vi "__FilterSet_CtrlEnable.vi"(4 "EIDRef 2":refnum<vi>[](array[refnum]), 6 "IDRef 2":refnum<vi>[](array[refnum]), 8 "error in (no error)":errorcluster, 9 "EIDRef":refnum<vi>[](array[refnum]), 10 "IDRef":refnum<vi>[](array[refnum]), 11 "CtrlRef":T1) -> (0 "error out":errorcluster)   [LabVIEW 2011]
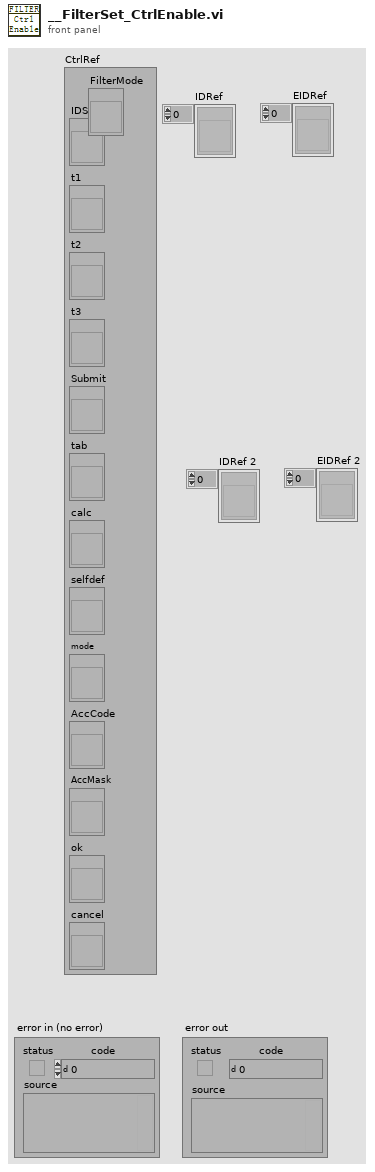
[diagram p1: front panel]
types:
  T1 = cluster{"FilterMode":refnum<vi>, "IDSet":refnum<vi>, "t1":refnum<vi>, "t2":refnum<vi>, "t3":refnum<vi>, "Submit":refnum<vi>, "tab":refnum<vi>, "calc":refnum<vi>, "selfdef":refnum<vi>, "mode":refnum<vi>, "AccCode":refnum<vi>, "AccMask":refnum<vi>, "ok":refnum<vi>, "cancel":refnum<vi>}
  T2 = enum16{"接收所有数据", "标准帧滤波（设定接收单个ID）", "扩展帧滤波（设定接收单个ID）", "标准帧滤波（仅ID，自由设定）", "扩展帧滤波（仅ID，自由设定）"}
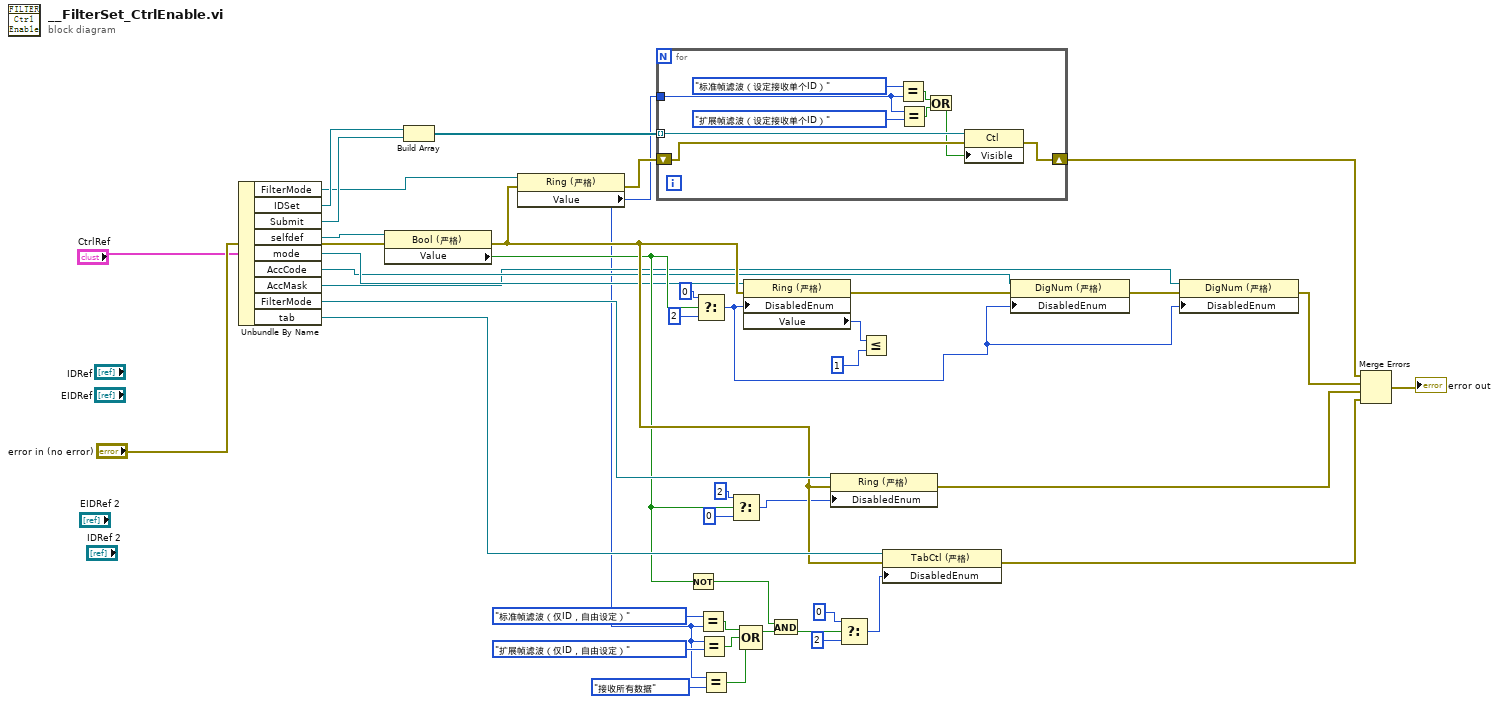
[diagram p0: block diagram]
diagram:
  n1 = Unbundle By Name("CtrlRef") -> ("FilterMode"=w38:refnum<vi>, "IDSet"=w41:refnum<vi>, "Submit"=w40:refnum<vi>, "selfdef"=w43:refnum<vi>, "mode"=w13:refnum<vi>, "AccCode"=w10:refnum<vi>, "AccMask"=w8:refnum<vi>, "FilterMode"=w32:refnum<vi>, "tab"=w31:refnum<vi>)
  n2 = property class="Bool (严格)"(reference=w43, error in="error in (no error)") -> (error out=w30:errorcluster, "Value"=w20:bool)  [unwired: 1 out]
  n3 = Build Array(w41, w40) -> (w39:refnum<vi>[])
  n4 = property class="Ring (严格)"(reference=w38, error in=w30) -> (error out=w37:errorcluster, "Value"=w3:u16)  [unwired: 1 out]
  n5 = for {
    tunnel: w39 -> [w52] mode=indexing
    shift-right: [w50] -> w36
    shift-left: w37 -> [w51]
    tunnel: w3 -> [w48]
    n6 = Equal?(x=T2."标准帧滤波（设定接收单个ID）", y=w48) -> (x = y?=w46:bool)
    n7 = Equal?(x=w48, y=T2."扩展帧滤波（设定接收单个ID）" ("x")) -> (x = y?=w45:bool)
    n8 = Or(x=w46, y=w45) -> (x .or. y?=w44:bool)
    n9 = property class="Ctl"(reference=w52, error in=w51, "Visible"=w44) -> (error out=w50:errorcluster)  [unwired: 1 out]
  }
  n10 = Not(x=w20) -> (.not. x?=w18:bool)
  n11 = Select(t=0, s=w20, f=2) -> (s? t:f=w1:i32)
  n12 = Equal?(x=T2."标准帧滤波（仅ID，自由设定）", y=w3) -> (x = y?=w27:bool)
  n13 = Equal?(x=w3, y=T2."扩展帧滤波（仅ID，自由设定）" ("x")) -> (x = y?=w5:bool)
  n14 = Equal?(x=w3, y=T2."接收所有数据") -> (x = y?=w4:bool)
  n15 = Select(t=2, s=w20, f=0) -> (s? t:f=w24:i32)
  n16 = Compound Arithmetic op=OR(w27, w5, w4) -> (w26:bool)
  n17 = property class="Ring (严格)"(reference=w13, error in=w30, "DisabledEnum"=w1) -> (error out=w11:errorcluster, "Value"=w12:u8)  [unwired: 1 out]
  n18 = And(x=w18, y=w26) -> (x .and. y?=w19:bool)
  n19 = property class="Ring (严格)"(reference=w32, error in=w30, "DisabledEnum"=w24) -> (error out=w42:errorcluster)  [unwired: 1 out]
  n20 = Select(t=0 ("f"), s=w19, f=2) -> (s? t:f=w22:i32)
  n21 = Less Or Equal?(x=w12, y=u8 1) -> ()  [unwired: 1 out]
  n22 = property class="TabCtl (严格)"(reference=w31, error in=w30, "DisabledEnum"=w22) -> (error out=w21:errorcluster)  [unwired: 1 out]
  n23 = property class="DigNum (严格)"(reference=w10, error in=w11, "DisabledEnum"=w1) -> (error out=w9:errorcluster)  [unwired: 1 out]
  n24 = property class="DigNum (严格)"(reference=w8, error in=w9, "DisabledEnum"=w1) -> (error out=w7:errorcluster)  [unwired: 1 out]
  n25 = Merge Errors(w36, w7, w42, w21) -> (→"error out":errorcluster)
